vi "CRIO_ReadAndParseTCP.vi"(8 "error in (no error)":errorcluster, 10 "Curr State":T1, 11 "TCP Network Connection in":refnum<k5>) -> (0 "error out":errorcluster, 1 "Update":bool, 2 "Command State":T1, 3 "TCP Network Connection out":refnum<k5>)   [LabVIEW 2017]
uses:
  CRIO_StateEnum.ctl
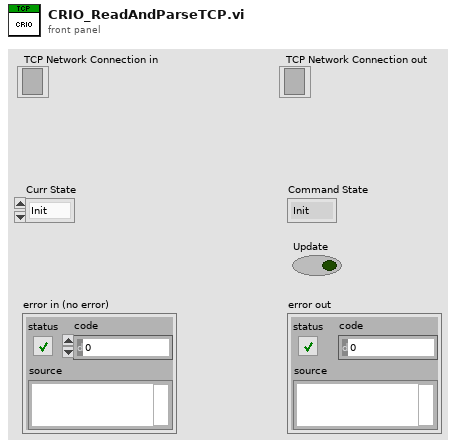
[diagram p1: front panel]
types:
  T1 = typedef "CRIO_StateEnum.ctl" = enum16{"Init", "Listen", "Wait", "Setup", "Ready to Launch", "Start Flight", "Accelerating", "Coasting", "Braking", "End Flight", "Loading", "Stop"}
  T2 = typedef "TCP_Read_Enum.ctl" = enum16{"No Data", "New Data", "No Connection"}
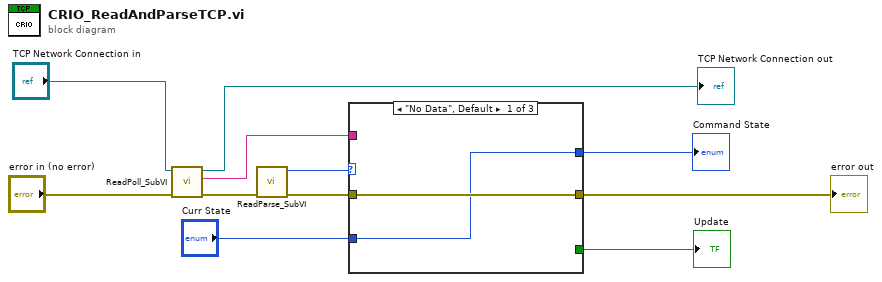
[diagram p0: block diagram]
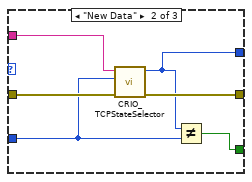
[diagram p2: hidden frame]
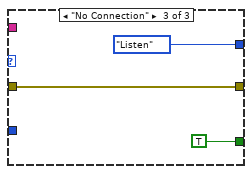
[diagram p3: hidden frame]
diagram:
  n1 = call "ReadPoll_SubVI.vi"("error in (no error)"="error in (no error)", "TCP Network Connection in"="TCP Network Connection in") -> ("error out"=w6:errorcluster, "data out"=w10:string, "TCP Network Connection out"=→"TCP Network Connection out":refnum<k5>)  [unwired: 7 in]
  n2 = call "ReadParse_SubVI.vi"("error in (no error)"=w6) -> ("Read Results"=w9:T2, "error out"=w7:errorcluster)  [unwired: 8 in]
  n3 = case shown="\"No Data\", Default" w9 {
    tunnel: [w13 w17 w22] -> w8
    tunnel: w7 -> [w13 w18 w22]
    tunnel: w10 -> [_ w19 _]
    tunnel: [w12 w15 CRIO_StateEnum."Listen" ("Command State")] -> w4
    tunnel: [_ w16 TRUE] -> w11
    tunnel: "Curr State" -> [w12 w14 _]
    frame "No Data", Default {
    }
    frame "New Data" {
      n4 = call "CRIO_TCPStateSelector.vi"("error in (no error)"=w18, "Curr State"=w14, "data in"=w19) -> ("error out"=w17:errorcluster, "Command State"=w15:T1)  [unwired: 7 in]
      n5 = Not Equal?(x=w15, y=w14) -> (x != y?=w16:bool)
    }
    frame "No Connection" {
    }
  }
  "Update" <- w11
  "Command State" <- w4
  "error out" <- w8
